vi "__init__.vi"(8 "error in":errorcluster, 10 "VISA resource name In":refnum<visa-resource-name>) -> (0 "error out":errorcluster, 3 "SR 830 & NI USB7855R out":refnum<class "SR 830 & NI USB7855R.lvclass">)   [LabVIEW 2020, in "SR 830 & NI USB7855R.lvclass"]
uses:
  SR 830 & NI USB7855R.lvclass
  SR 830 & NI USB7855R.lvclass/SR 830 & NI USB7855R.ctl
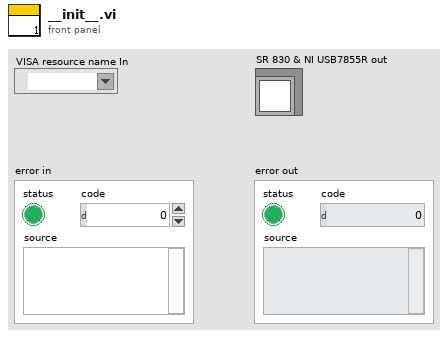
[diagram p1: front panel]
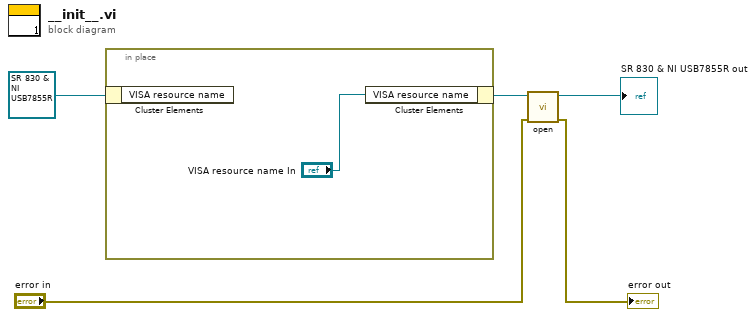
[diagram p0: block diagram]
diagram:
  n1 = in-place {
    n2 = in-place-cluster #1(refnum<class "SR 830 & NI USB7855R.lvclass"> refnum ("SR 830 & NI USB7855R.lvclass")) -> ()  [unwired: 1 out]
    n3 = in-place-cluster #1("VISA resource name"="VISA resource name In") -> (w4:refnum<class "SR 830 & NI USB7855R.lvclass">)
  }
  n4 = call-dynamic "open.vi"("error in (no error)"="error in", "Instrument in"=w4) -> ("error out"=→"error out":errorcluster, "Instrument out"=→"SR 830 & NI USB7855R out":refnum<class "SR 830 & NI USB7855R.lvclass">)  [unwired: 8 in]
